vi "WriteTableToCalibrationVolumes.vi"(11 "NewVal":string[][](array[string])) -> ()   [LabVIEW 2012]
uses:
  GlobalVariables/CalibrationVolumes.vi
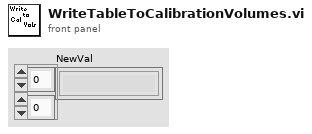
[diagram p1: front panel]
types:
  T1 = cluster{"CalibrationVolumes":dbl[], "SetName":string}[]
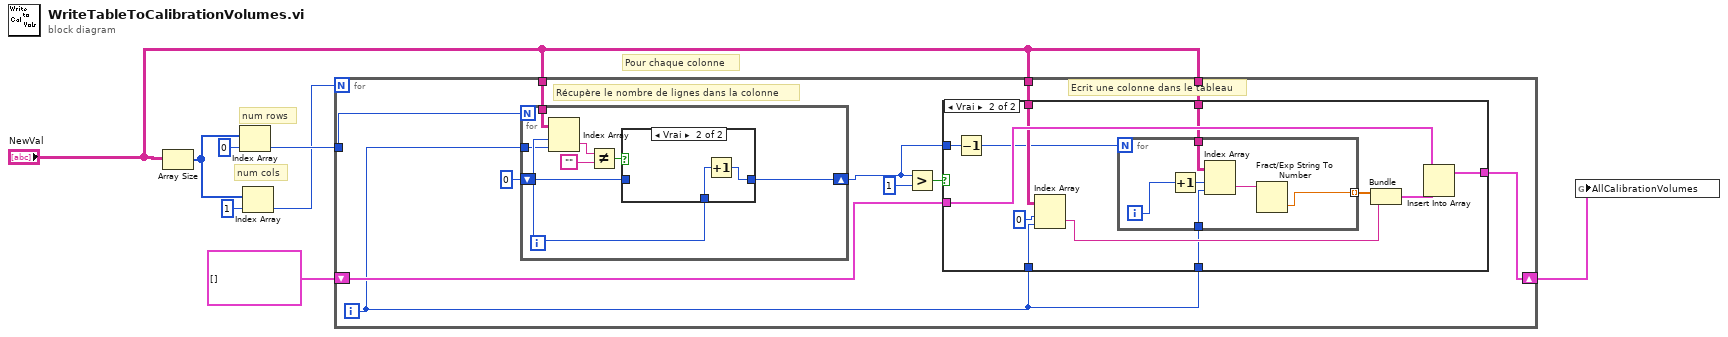
[diagram p0: block diagram]
diagram:
  # "Pour chaque colonne"
  # "num cols"
  # "num rows"
  n1 = Array Size(array="NewVal") -> (size(s)=w2:i32[])
  n2 = Index Array(array=w2, index=0) -> (element=w5:i32)
  n3 = Index Array(array=w2, index=1) -> (element=w4:i32)
  n4 = for {
    N: w4 -> [_]
    tunnel: w5 -> [w19]
    tunnel: "NewVal" -> [w17]
    shift-right: [w13] -> w6
    shift-left: T1 [] ("AllCalibrationVolumes") -> [w14]
    tunnel: "NewVal" -> [w12]
    tunnel: "NewVal" -> [w9]
    i -> [w10]
    # "Ecrit une colonne dans le tableau"
    # "Récupère le nombre de lignes dans la colonne"
    n5 = for {
      N: w19 -> [_]
      shift-right: [w45] -> w11
      shift-left: 0 -> [w46]
      tunnel: w17 -> [w41]
      tunnel: w10 -> [w39]
      i -> [w40]
      n6 = Index Array(array=w41, index (row)=w40, index (col)=w39) -> (element=w43:string)
      n7 = Not Equal?(x=w43, y="") -> (x != y?=w44:bool)
      n8 = case shown="Vrai" w44 {
        tunnel: w46 -> [w47 _]
        tunnel: [w47 w48] -> w45
        tunnel: w40 -> [_ w49]
        frame False {
        }
        frame True {
          n9 = Increment(x=w49) -> (x+1=w48:i32)
        }
      }
    }
    n10 = Greater?(x=w11, y=1) -> (0:w16:bool)
    n11 = case shown="Vrai" w16 {
      tunnel: w14 -> [w20 w32]
      tunnel: [w20 w31] -> w13
      tunnel: w12 -> [_ w29]
      tunnel: w10 -> [_ w27]
      tunnel: w11 -> [_ w22]
      tunnel: w10 -> [_ w25]
      tunnel: w9 -> [_ w24]
      frame False {
      }
      frame True {
        n12 = Decrement(x=w22) -> (x-1=w21:i32)
        n13 = Index Array(array=w29, index (row)=0, index (col)=w27) -> (element=w26:string)
        n14 = for {
          N: w21 -> [_]
          tunnel: w25 -> [w38]
          tunnel: w24 -> [w35]
          tunnel: [w33] -> w23 mode=indexing
          i -> [w36]
          n15 = Increment(x=w36) -> (x+1=w37:i32)
          n16 = Index Array(array=w35, index (row)=w37, index (col)=w38) -> (element=w34:string)
          n17 = Fract/Exp String To Number(string=w34) -> (number=w33:dbl)  [unwired: 3 in, 1 out]
        }
        n18 = Bundle(w23, w26) -> (w30:cluster{dbl[], string})  [unwired: 1 in]
        n19 = Insert Into Array(array=w32, new element=w30) -> (w31:T1)  [unwired: 1 in]
      }
    }
  }
  n20 = global write "CalibrationVolumes.vi" "AllCalibrationVolumes"(w6) -> ()
